vi "CreateNewImage.vi"(8 "Error In":errorcluster, 9 "Display Image In":T1, 10 "Image Name":string, 11 "Original Image":T1) -> (0 "Error Out":errorcluster, 2 "Image Type":T2 items=["Grayscale (U8)", "Grayscale (I16)", "Grayscale (SGL)", "Complex (CSG)", "RGB (U32)", "HSL (U32)", "RGB (U64)", "Grayscale (U16)"], 3 "Orignal Image Temp Out":T1)   [LabVIEW 2019]
uses:
  <vilib>/vision/Image Controls.llb/IMAQ Image.ctl
panel:
  out "Image":T1(plugin-control)
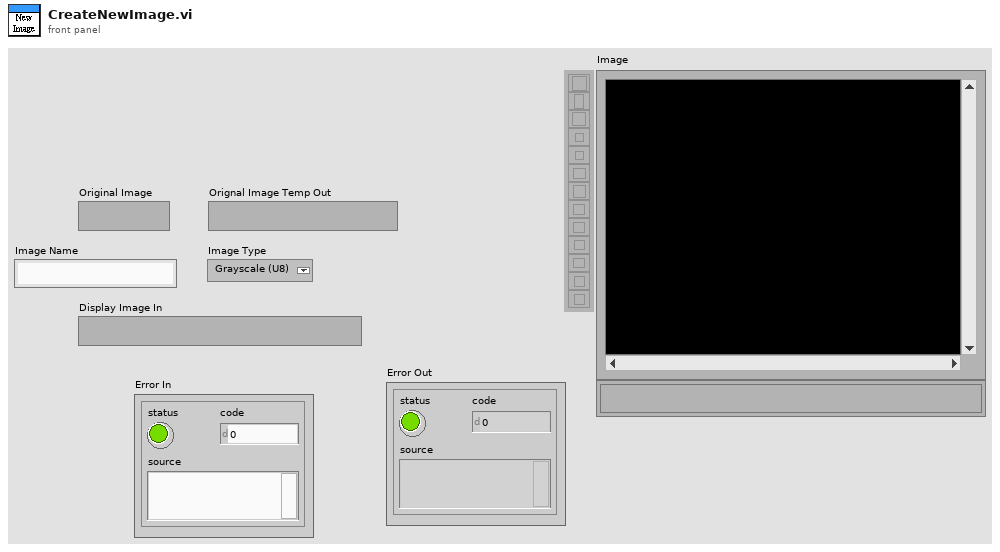
[diagram p1: front panel]
types:
  T1 = typedef "IMAQ Image.ctl" = refnum<image>
  T2 = typedef "Image Type" = u32
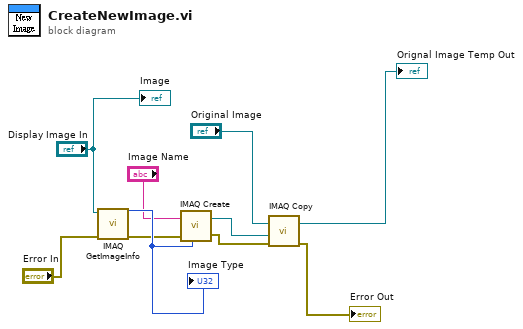
[diagram p0: block diagram]
diagram:
  n1 = call "IMAQ GetImageInfo"("error in (no error)"="Error In", "Image"="Display Image In") -> ("error out"=w4:errorcluster, "Image Type"=w9:T2)  [unwired: 2 in, 6 out]
  "Image Type" <- w9
  n2 = call "IMAQ Create"("Image Name"="Image Name", "Image Type"=w9, "error in (no error)"=w4) -> ("New Image"=w6:T1, "error out"=w3:errorcluster)  [unwired: 2 in]
  n3 = call "IMAQ Copy"("error in (no error)"=w3, "Image Dst"=w6, "Image Src"="Original Image") -> ("error out"=→"Error Out":errorcluster, "Image Dst Out"=→"Orignal Image Temp Out":T1)  [unwired: 3 in]
  "Image" <- "Display Image In"
